vi "InitializeRG.vi"(0 "VISA resource name":refnum<visa-resource-name>, 1 "timeout (10sec)":u32=10000) -> (2 "VISA resource name out":refnum<visa-resource-name>, 3 "return count":u32, 4 "return count 2":u32, 5 "error out":errorcluster)   [LabVIEW 2009]
uses:
  <vilib>/Instr/_visa.llb/VISA Configure Serial Port (Instr).vi
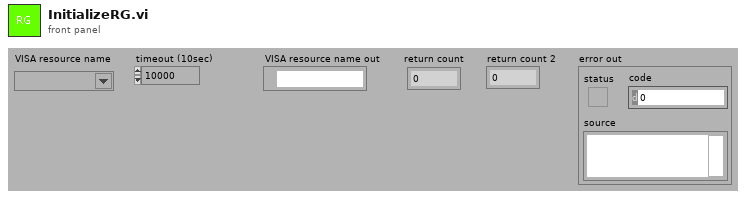
[diagram p1: front panel]
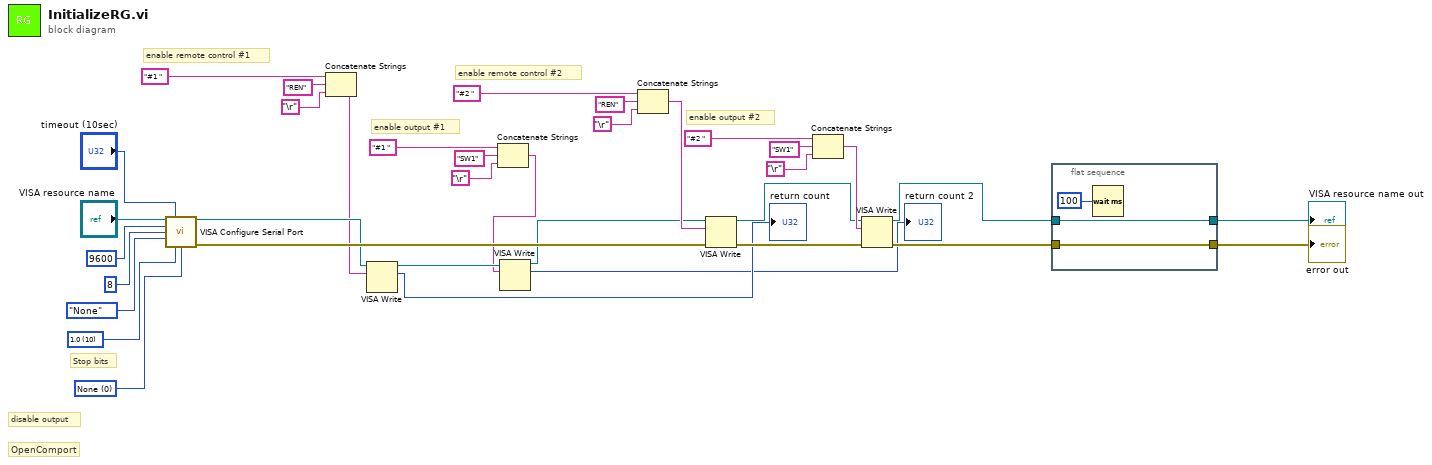
[diagram p0: block diagram]
diagram:
  w24 = u16 0 items=["None", "XON/XOFF", "RTS/CTS", "XON/XOFF & RTS/CTS", "DTR/DSR", "XON/XOFF & DTR/DSR"] ("flow control (0:none)")
  w23 = u16 10 items=["1.0"=10, "1.5"=15, "2.0"=20] ("stop bits (10: 1 bit)")
  # "enable output #1"
  # "enable remote control #1"
  # "OpenComport"
  # "Stop bits"
  # "enable remote control #2"
  # "enable output #2"
  # "disable output"
  n1 = call-poly "VISA Configure Serial Port"("VISA resource name"="VISA resource name", "timeout (10sec)"="timeout (10sec)", "baud rate (9600)"=u32 9600, "data bits (8)"=u16 8, "parity (0:none)"=enum16{"None", "Odd", "Even", "Mark", "Space"}."None", "stop bits (10: 1 bit)"=w23, "flow control (0:none)"=w24) -> ("VISA resource name out"=w13:refnum<visa-resource-name>, "error out"=w29:errorcluster)  [unwired: 7 in]
  n2 = Concatenate Strings("#1 " ("initial string"), "REN" ("string"), "\r") -> (w7:string)
  n3 = VISA Write(VISA resource name=w13, write buffer=w7) -> (VISA resource name out=w12:refnum<visa-resource-name>, return count=→"return count":u32)  [unwired: 1 in, 1 out]
  n4 = Concatenate Strings("#1 " ("format string"), "SW1" ("initial string"), "\r" ("input 1")) -> (w3:string)
  n5 = VISA Write(VISA resource name=w12, write buffer=w3) -> (VISA resource name out=w11:refnum<visa-resource-name>, return count=→"return count 2":u32)  [unwired: 1 in, 1 out]
  n6 = Concatenate Strings("#2 " ("initial string"), "REN" ("string"), "\r") -> (w27:string)
  n7 = VISA Write(VISA resource name=w11, write buffer=w27, error in (no error)=w29) -> (VISA resource name out=w25:refnum<visa-resource-name>, error out=w26:errorcluster)  [unwired: 1 out]
  n8 = Concatenate Strings("#2 " ("format string"), "SW1" ("initial string"), "\r" ("input 1")) -> (w28:string)
  n9 = VISA Write(VISA resource name=w25, write buffer=w28, error in (no error)=w26) -> (VISA resource name out=w33:refnum<visa-resource-name>, error out=w32:errorcluster)  [unwired: 1 out]
  n10 = flat-sequence {
    tunnel: w33 -> [w36]
    tunnel: w32 -> [w37]
    tunnel: [w37] -> w35
    tunnel: [w36] -> w34
    frame #0 {
      n11 = Wait (ms)(milliseconds to wait=u32 100) -> ()  [unwired: 1 out]
    }
  }
  "error out" <- w35
  "VISA resource name out" <- w34
